vi "FL Create Membership Function.vi"   [LabVIEW 2017, in "NI_Fuzzy_Logic_API.lvlib"]
doc: "Creates a membership function for a linguistic variable. You also can use the Define Variable dialog box to create membership functions interactively."
uses:
  <vilib>/addons/Fuzzy Logic/NI_Fuzzy_Logic_API.lvlib
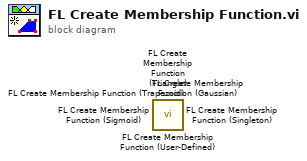
[diagram p0: block diagram]
diagram:
  n1 = call <vilib>:"FL Create Membership Function (User-Defined).vi"() -> ()  [unwired: 14 in, 2 out]
  n2 = call <vilib>:"FL Create Membership Function (Gaussian).vi"() -> ()  [unwired: 14 in, 2 out]
  n3 = call <vilib>:"FL Create Membership Function (Sigmoid).vi"() -> ()  [unwired: 14 in, 2 out]
  n4 = call <vilib>:"FL Create Membership Function (Singleton).vi"() -> ()  [unwired: 14 in, 2 out]
  n5 = call <vilib>:"FL Create Membership Function (Trapezoid).vi"() -> ()  [unwired: 14 in, 2 out]
  n6 = call <vilib>:"FL Create Membership Function (Triangle).vi"() -> ()  [unwired: 14 in, 2 out]
